vi "IMAQ_overlay_points_extrinsic.vi"(10 "array":cluster{"X":i32, "Y":i32}[](array[cluster]), 11 "extrinsic":cluster{"extrinsic":dbl[][], "resolution":i32[]}) -> (3 "new array":cluster{"X":i32, "Y":i32}[](array[cluster]))   [LabVIEW 2017]
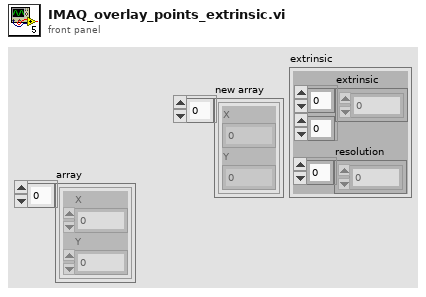
[diagram p1: front panel]
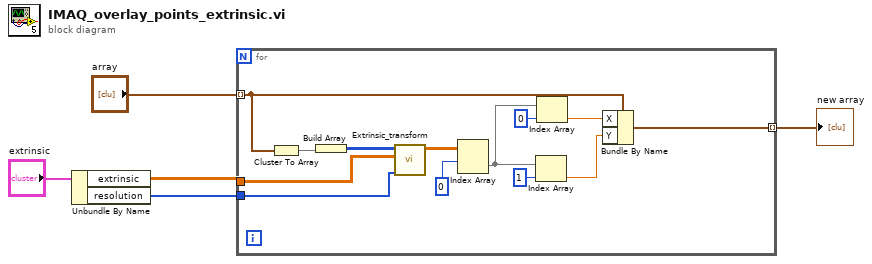
[diagram p0: block diagram]
diagram:
  n1 = Unbundle By Name("extrinsic") -> ("extrinsic"=w2:dbl[][], "resolution"=w1:i32[])
  n2 = for {
    tunnel: w2 -> [w16]
    tunnel: "array" -> [w13] mode=indexing
    tunnel: [w7] -> w4 mode=indexing
    tunnel: w1 -> [w6]
    n3 = Cluster To Array(cluster=w13) -> (array=w18:i32[])
    n4 = Build Array(w18) -> (w17:i32[][])
    n5 = call "Extrinsic_transform.vi"("resolution"=w6, "extrinsic"=w16, "X"=w17) -> ("X'"=w15:dbl[][])  [unwired: 8 in]
    n6 = Index Array(array=w15, index (row)=0) -> (element=w9:dbl[])  [unwired: 1 in]
    n7 = Index Array(array=w9, index=1) -> (element=w8:dbl)
    n8 = Index Array(array=w9, index=0) -> (element=w12:dbl)
    n9 = Bundle By Name(cluster=w13, "X"=w12, "Y"=w8) -> (w7:cluster{"X":i32, "Y":i32})
  }
  "new array" <- w4
